vi "Delete Endpoint.vi"(8 "error in (no error)":errorcluster, 11 "Endpoint":refnum<class "Endpoint.lvclass">) -> (0 "error out":errorcluster)   [LabVIEW 2015, in "NI_AWS_SNS.lvlib" / "Endpoint.lvclass"]
uses:
  Endpoint.lvclass
  Core/ARN/ARN.lvclass
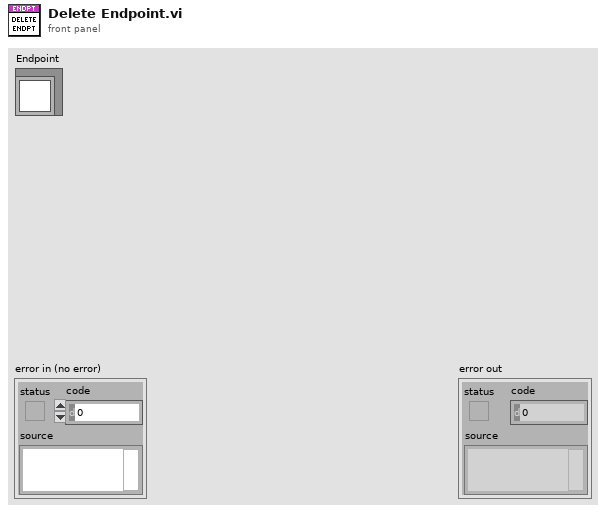
[diagram p1: front panel]
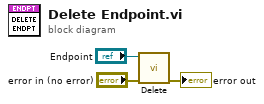
[diagram p0: block diagram]
diagram:
  n1 = call "Delete.vi"("error in (no error)"="error in (no error)", "ARN in"="Endpoint") -> ("error out"=→"error out":errorcluster)  [unwired: 9 in]
